vi "Write SP.vi"(8 "error in (no error)":errorcluster, 10 "SP":dbl, 11 "Update Device Setpoint in":refnum<class "Update Device Setpoint.lvclass">) -> (0 "error out":errorcluster, 3 "Update Device Setpoint out":refnum<class "Update Device Setpoint.lvclass">)   [LabVIEW 2014, in "Controller.lvlib" / "Update Device Setpoint.lvclass"]
uses:
  Update Device Setpoint.lvclass
  Update Device Setpoint.lvclass/Update Device Setpoint.ctl
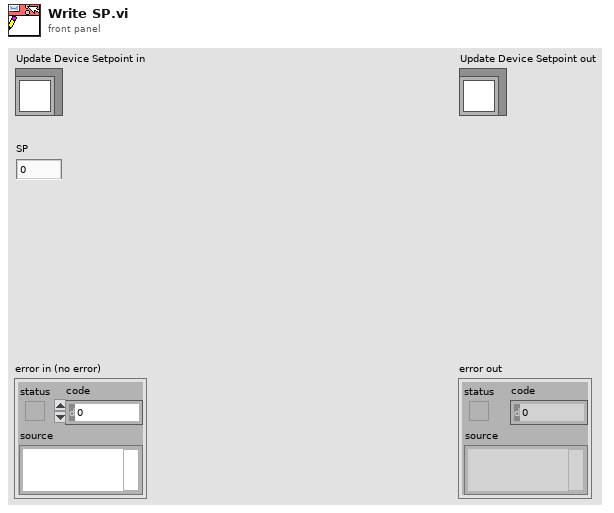
[diagram p1: front panel]
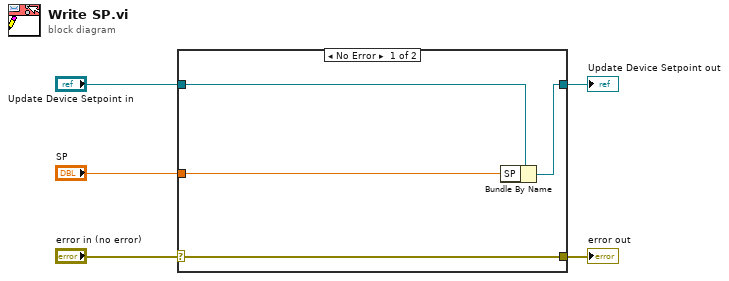
[diagram p0: block diagram]
diagram:
  n1 = case shown="No Error" "error in (no error)" {
    selector: "error in (no error)" -> [w9 w10]
    tunnel: [w9 w10] -> w4
    tunnel: [w7 w11] -> w2
    tunnel: "Update Device Setpoint in" -> [w8 w11]
    tunnel: "SP" -> [w6 _]
    frame No Error {
      n2 = Bundle By Name(cluster=w8, "SP"=w6) -> (w7:refnum<class "Update Device Setpoint.lvclass">)
    }
    frame Error {
    }
  }
  "error out" <- w4
  "Update Device Setpoint out" <- w2
